vi "r09543017.vi"() -> ()   [LabVIEW 2014]
uses:
  subvi/EyeOptionsCluster.ctl
  <vilib>/userdefined/High Color/IMAQdx.ctl
  <vilib>/vision/NI_Vision_Development_Module.lvlib
  <vilib>/vision/driver/NI_Vision_Acquisition_Software.lvlib
panel:
  in  "Options":T1={"Level"=4, "Max. Iterations"=5, "Window Size"=17, "Displacement Threshold"=0.01}
  out "Cluster":cluster{dbl, dbl}
  in  "Stop":bool
  out "Image":T2(plugin-control)
  in  "Eye Options":T3={"Eye Size"=1.0, "Overlay Eyes?"=TRUE, "Eye Tracking?"=TRUE} {"Eye Size" items=["Small"=0.5, "Medium"=1, "Large"=2]}
  in  "Select Points":bool
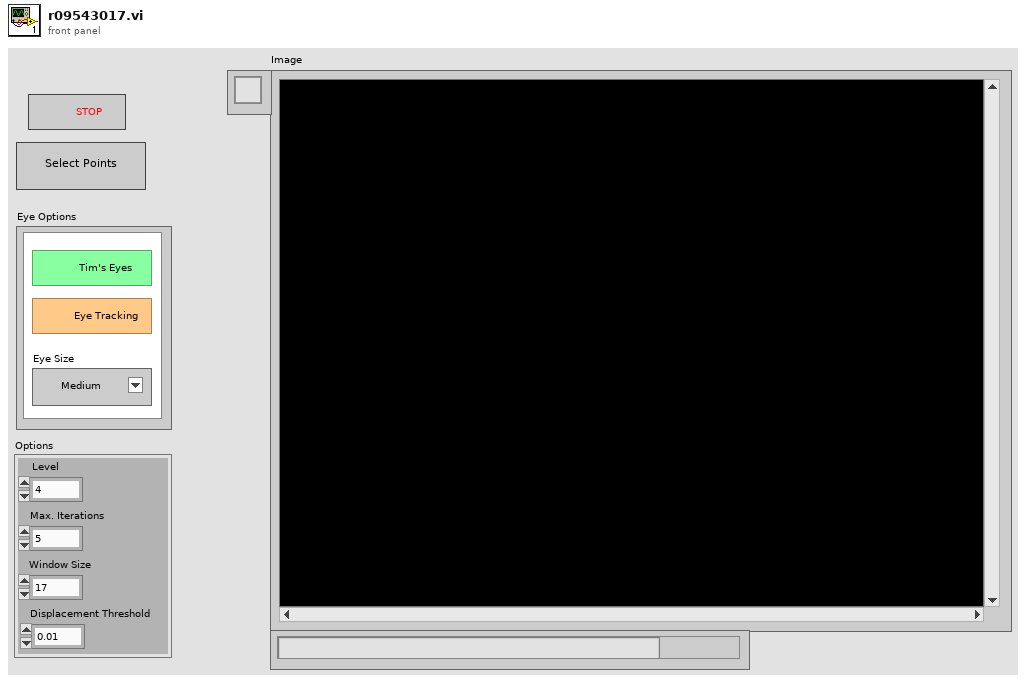
[diagram p1: front panel]
types:
  T1 = cluster{"Level":i32, "Max. Iterations":i32, "Window Size":i32, "Displacement Threshold":dbl}
  T2 = typedef "IMAQ Image.ctl" = refnum<image>
  T3 = typedef "EyeOptionsCluster.ctl" = cluster{"Eye Size":sgl, "Overlay Eyes?":bool, "Eye Tracking?":bool}
  T4 = typedef "IMAQdx.ctl" = refnum<k21>
  T5 = cluster{"Global Rectangle":i32[], "Contours":cluster{"Contour Type":u32, "ROI Type":u32, "Points":i32[]}[]}
  T6 = typedef "ROI Descriptor" = cluster{"Global Rectangle":i32[], "Contours":cluster{"ID":enum32{"External", "Internal"}, "Type":u32, "Coordinates":i32[]}[]}
  T7 = typedef "IMAQ Point" = cluster{"X":sgl, "Y":sgl}
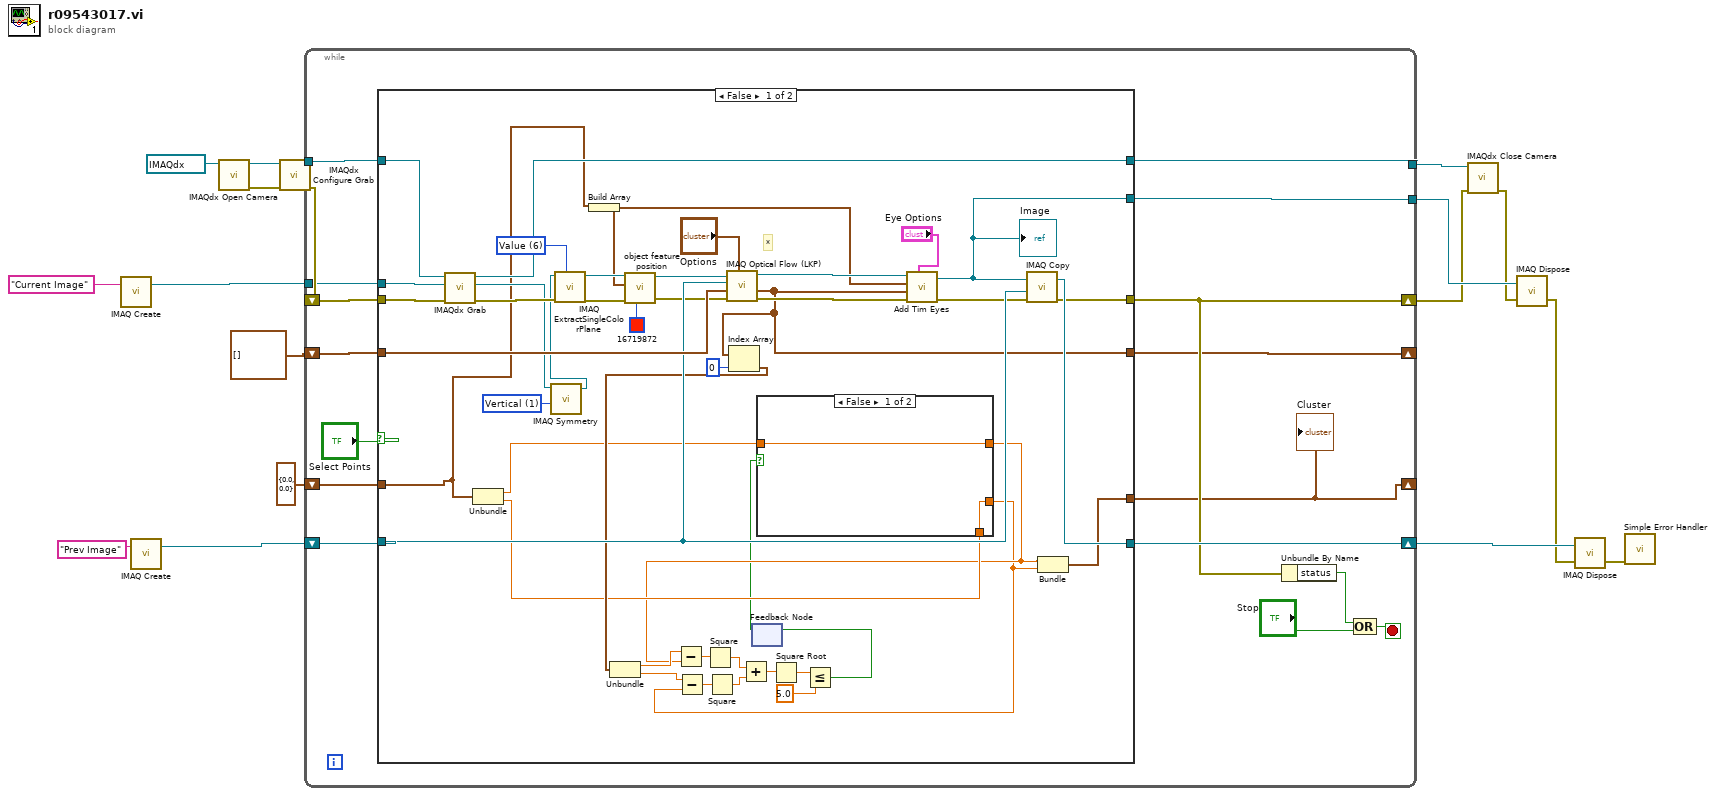
[diagram p0: block diagram]
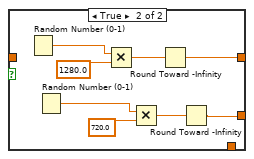
[diagram p2: hidden frame]
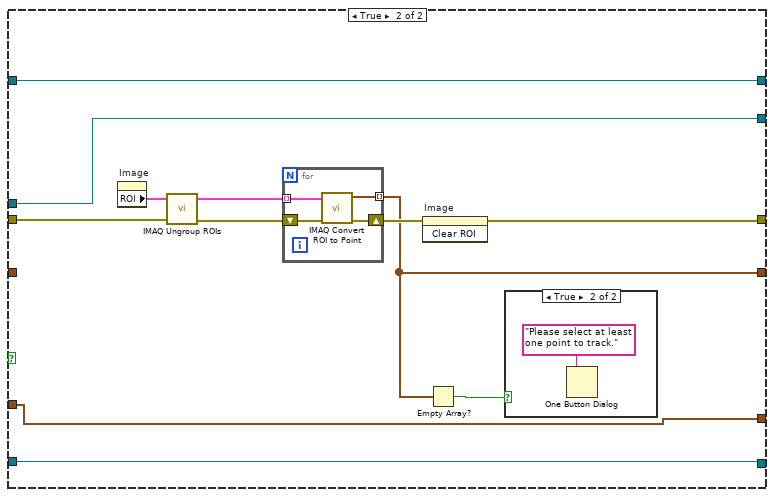
[diagram p3: hidden frame]
diagram:
  n1 = call "IMAQ Create"("Image Name"="Current Image") -> ("New Image"=w3:T2)  [unwired: 3 in, 2 out]
  n2 = call "IMAQ Create"("Image Name"="Prev Image") -> ("New Image"=w2:T2)  [unwired: 3 in, 2 out]
  n3 = call <vilib>:"IMAQdx Open Camera.vi"("Session In"=T4 "cam0") -> ("error out"=w11:errorcluster, "Session Out"=w12:T4)  [unwired: 9 in]
  n4 = call <vilib>:"IMAQdx Configure Grab.vi"("error in"=w11, "Session In"=w12) -> ("error out"=w4:errorcluster, "Session Out"=w5:T4)  [unwired: 8 in]
  n5 = while {
    tunnel: w3 -> [w24]
    shift-right: [w29] -> w15
    shift-left: w2 -> [w31]
    shift-right: [w26] -> _
    shift-left: cluster{"X":sgl, "Y":sgl}[] [] ("Feature Points Out") -> [w27]
    shift-right: [w28] -> w9
    shift-left: w4 -> [w34]
    tunnel: [w23] -> w16
    tunnel: w5 -> [w22]
    tunnel: [w21] -> w14
    shift-right: [w20] -> _
    shift-left: cluster{dbl, dbl} {0.0, 0.0} -> [w19]
    stop <- w32 stop-if-true
    n6 = case shown="False" "Select Points" {
      tunnel: w34 -> [w79 w96]
      tunnel: w24 -> [w78 w95]
      tunnel: w31 -> [w72 w101]
      tunnel: [w77 w101] -> w29
      tunnel: [w76 w92] -> w28
      tunnel: w27 -> [w75 _]
      tunnel: [w56 w94] -> w26
      tunnel: [w66 w95] -> w23
      tunnel: w22 -> [w74 w91]
      tunnel: [w73 w91] -> w21
      tunnel: [w53 w90] -> w20
      tunnel: w19 -> [w52 w90]
      frame False {
        w48 = 6 items=["Red", "Green", "Blue", "Hue", "Saturation", "Luminance", "Value", "Intensity"] ("Color Plane")
        w57 = u32 1 items=["Horizontal", "Vertical", "Central", "1st Diagonal", "2nd Diagonal"] ("Type of Symmetry")
        # "*"
        n7 = call <vilib>:"IMAQdx Grab.vi"("error in"=w79, "Image In"=w78, "Session In"=w74) -> ("error out"=w70:errorcluster, "Image Out"=w59:T2, "Session Out"=w73:T4)  [unwired: 5 in, 1 out]
        n8 = Unbundle(w52) -> (w51:dbl, w50:dbl)
        n9 = call "IMAQ Symmetry"("Type of Symmetry"=w57, "Image Src"=w59) -> ("Image Dst Out"=w58:T2)  [unwired: 3 in, 1 out]
        n10 = call "IMAQ ExtractSingleColorPlane"("Color Plane"=w48, "error in (no error)"=w70, "Image Src"=w58) -> ("error out"=w64:errorcluster, "Image Dst Out"=w68:T2)  [unwired: 7 in]
        n11 = Build Array(w52) -> (w62:cluster{dbl, dbl}[])
        n12 = call "object feature position.vi"("Color"=u32 16719872, "Error In"=w64, "Feature Ponts"=w62, "Image"=w68) -> ("Error Out"=w61:errorcluster, "Image Out"=w67:T2)  [unwired: 6 in]
        n13 = call "IMAQ Optical Flow (LKP)"("Options"="Options", "error in (no error)"=w61, "Feature Points In"=w75, "Previous Frame"=w72, "Current Frame"=w67) -> ("error out"=w69:errorcluster, "Feature Points Out"=w56:cluster{"X":sgl, "Y":sgl}[], "Current Frame Out (dup)"=w65:T2)  [unwired: 1 in, 3 out]
        n14 = Index Array(array=w56, index=0) -> (element=w54:cluster{"X":sgl, "Y":sgl})
        n15 = Unbundle(w54) -> ("X"=w47:sgl, "Y"=w45:sgl)
        n16 = feedback #1() -> (w35:bool)  [unwired: 1 in]
        n17 = case shown="False" w35 {
          tunnel: [w80 w84] -> w46
          tunnel: [w81 w82] -> w44
          tunnel: w50 -> [w81 _]
          tunnel: w51 -> [w80 _]
          frame False {
          }
          frame True {
            n18 = Random Number (0-1)() -> (number: 0 to 1=w89:dbl)
            n19 = Random Number (0-1)() -> (number: 0 to 1=w86:dbl)
            n20 = Multiply(x=w89, y=1280.0) -> (x*y=w85:dbl)
            n21 = Multiply(x=w86, y=720.0) -> (x*y=w83:dbl)
            n22 = Round Toward -Infinity(1:w85) -> (0:w84:dbl)
            n23 = Round Toward -Infinity(1:w83) -> (0:w82:dbl)
          }
        }
        n24 = Subtract(x=w47, y=w46) -> (x-y=w43:dbl)
        n25 = Subtract(x=w45, y=w44) -> (x-y=w42:dbl)
        n26 = Square(x=w43) -> (x^2=w41:dbl)
        n27 = Square(x=w42) -> (x^2=w40:dbl)
        n28 = Add(x=w41, y=w40) -> (x+y=w39:dbl)
        n29 = Square Root(x=w39) -> (sqrt(x)=w38:dbl)
        n30 = Less Or Equal?(x=w38, y=5.0) -> (x <= y?=w36:bool)
        n31 = feedback-in #1(w36) -> ()
        n32 = call "Add Tim Eyes.vi"("Options"="Eye Options", "error in (no error)"=w69, "Eye Coordinates"=w56, "Feature Coordinates"=w62, "ImageRef In"=w65) -> ("error out"=w71:errorcluster, "ImageRef out"=w66:T2)  [unwired: 5 in]
        "Image" <- w66
        n33 = call "IMAQ Copy"("error in (no error)"=w71, "Image Dst"=w72, "Image Src"=w66) -> ("error out"=w76:errorcluster, "Image Dst Out"=w77:T2)  [unwired: 3 out]
        n34 = Bundle(w46, w44) -> (w53:cluster{dbl, dbl})  [unwired: 1 in]
      }
      frame True {
        # "When user selects new points on image, create one of more ROI (region of interest) and feed them to a shift register, so they can be accessed in subsequent loops"
        n35 = property on="Image" class="ImageControl"() -> ("ROI"=w100:T5)  [unwired: 2 in, 2 out]
        n36 = call "IMAQ Ungroup ROIs"("error in (no error)"=w96, "ROI Descriptor"=w100) -> ("error out"=w99:errorcluster, "ROI Descriptors out"=w98:T6[])  [unwired: 2 out]
        n37 = for {
          shift-right: [w103] -> w97
          shift-left: w99 -> [w106]
          tunnel: w98 -> [w105] mode=indexing
          tunnel: [w104] -> w94 mode=indexing
          n38 = call "IMAQ Convert ROI to Point"("error in (no error)"=w106, "ROI Descriptor"=w105) -> ("error out"=w103:errorcluster, "Point"=w104:T7)  [unwired: 7 out]
        }
        n39 = invoke on="Image" class="ImageControl" method="Clear ROI"(error in=w97) -> (error out=w92:errorcluster)  [unwired: 2 in, 2 out]
        n40 = Empty Array?(array=w94) -> (empty?=w93:bool)
        n41 = case shown="True" w93 {
          frame False {
          }
          frame True {
            n42 = One Button Dialog(message="Please select at least one point to track.") -> ()  [unwired: 2 out]
          }
        }
      }
    }
    "Cluster" <- w20
    n43 = Unbundle By Name(w28) -> ("status"=w30:bool)
    n44 = Compound Arithmetic op=OR(w30, "Stop") -> (w32:bool)
  }
  n45 = call <vilib>:"IMAQdx Close Camera.vi"("error in"=w9, "Session In"=w14) -> ("error out"=w8:errorcluster)  [unwired: 9 in]
  n46 = call "IMAQ Dispose"("Image"=w16, "error in (no error)"=w8) -> ("error out"=w7:errorcluster)  [unwired: 1 in, 3 out]
  n47 = call "IMAQ Dispose"("Image"=w15, "error in (no error)"=w7) -> ("error out"=w6:errorcluster)  [unwired: 1 in, 3 out]
  n48 = call <vilib>:"Simple Error Handler.vi"("error in (no error)"=w6) -> ()  [unwired: 1 in, 8 out]
